vi "write positions to cvt or reload pico.vi"(8 "error in (no error)":errorcluster, 10 "Array":dbl[](array[numeric]), 11 "Picomotor8742dotNet in":refnum<class "Picomotor8742dotNet.lvclass">) -> (0 "error out":errorcluster, 2 "new command":string, 3 "Picomotor8742dotNet out":refnum<class "Picomotor8742dotNet.lvclass">)   [LabVIEW 2020, in "Picomotor8742dotNet.lvclass"]
uses:
  Picomotor8742dotNet.lvclass
  Picomotor8742dotNet.lvclass/Picomotor8742dotNet.ctl
  shared/CompressAndUpdate(Poly)/CompressAndUpdate(Numeric).vi
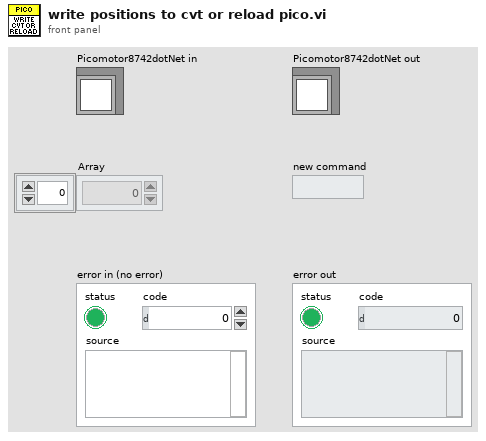
[diagram p1: front panel]
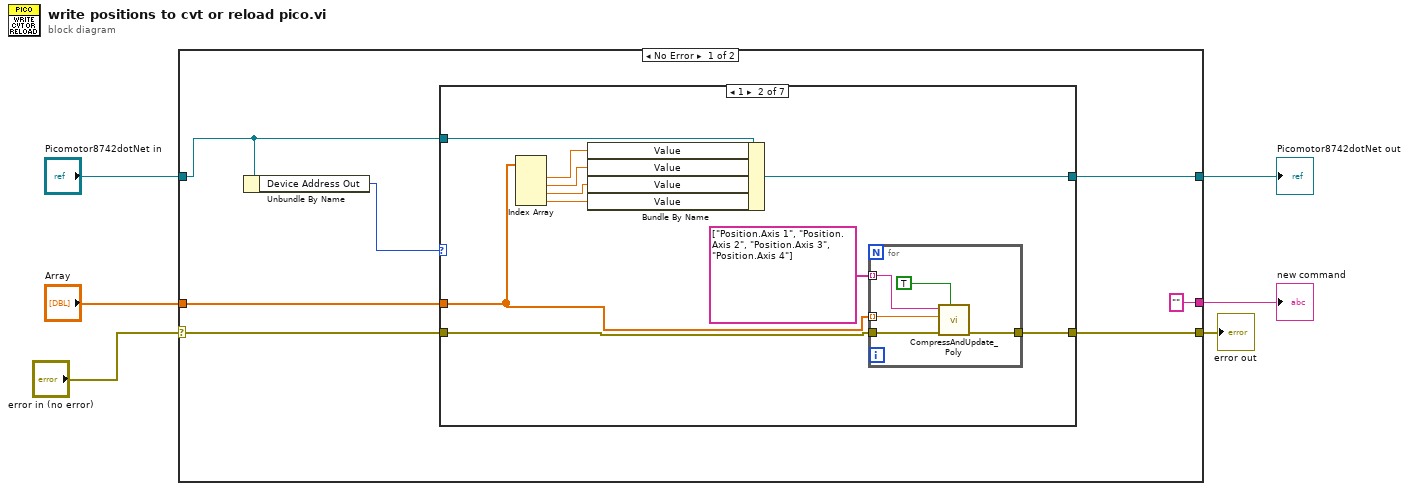
[diagram p0: block diagram]
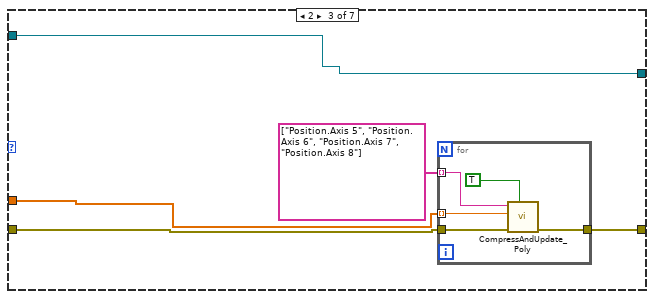
[diagram p3: hidden frame]
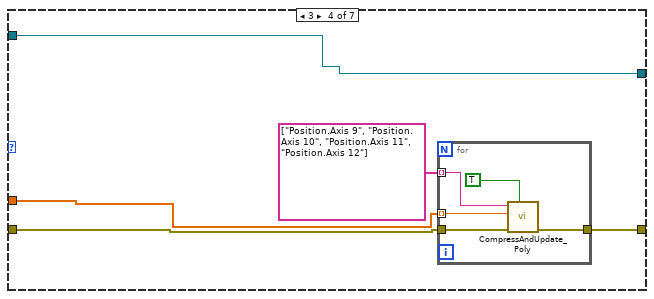
[diagram p4: hidden frame]
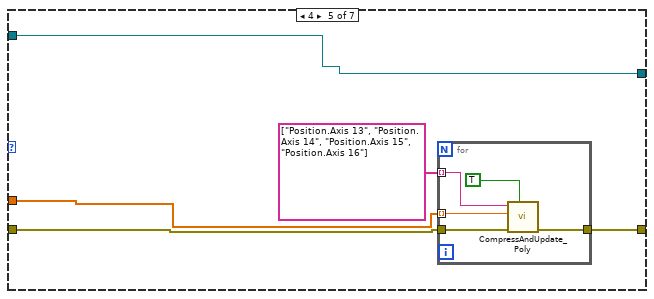
[diagram p5: hidden frame]
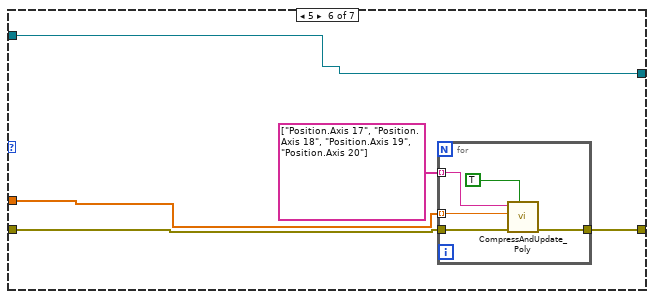
[diagram p6: hidden frame]
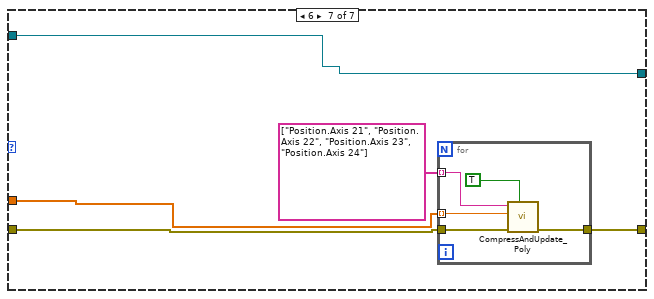
[diagram p7: hidden frame]
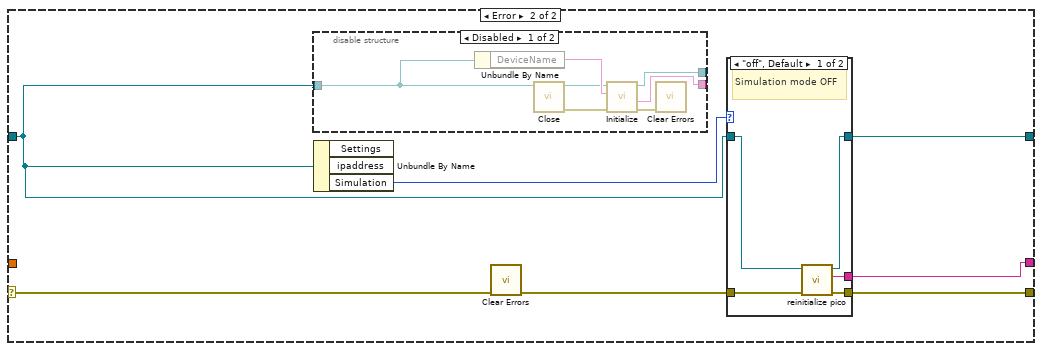
[diagram p8: hidden frame]
diagram:
  n1 = case shown="No Error" "error in (no error)" {
    selector: "error in (no error)" -> [w12 w86]
    tunnel: "Array" -> [w11 _]
    tunnel: [w13 w87] -> w2
    tunnel: "Picomotor8742dotNet in" -> [w8 w82]
    tunnel: [w10 w84] -> w4
    tunnel: ["" ("new command") w83] -> w5
    frame No Error {
      n2 = Unbundle By Name(w8) -> ("Device Address Out"=w7:i32)
      n3 = case shown="1" w7 {
        tunnel: [w14 w24 w34 w44 w54 w64 w74] -> w13
        tunnel: w12 -> [w14 w23 w33 w43 w53 w63 w73]
        tunnel: w11 -> [_ w18 w32 w42 w52 w62 w72]
        tunnel: [w15 w17 w31 w41 w51 w61 w71] -> w10
        tunnel: w8 -> [w15 w16 w31 w41 w51 w61 w71]
        frame 0, Default {
        }
        frame 1 {
          n4 = Index Array(array=w18) -> (element #1=w19:dbl, element #2=w20:dbl, element #3=w21:dbl, element #4=w22:dbl)  [unwired: 4 in]
          n5 = Bundle By Name(cluster=w16, "Value"=w19, "Value"=w20, "Value"=w21, "Value"=w22) -> (w17:refnum<class "Picomotor8742dotNet.lvclass">)
          n6 = for {
            tunnel: w18 -> [w28] mode=indexing
            tunnel: string[] ["Position.Axis 1", "Position.Axis 2", "Position.Axis 3", "Position.Axis 4"] -> [w29] mode=indexing
            tunnel: w23 -> [w27]
            tunnel: [w26] -> w24
            n7 = call-poly "CompressAndUpdate_Poly.vi"("force CVT update (false)"=TRUE ("force CVT update"), "error in"=w27, "Numeric"=w28, "command or variable name"=w29) -> ("error out"=w26:errorcluster)  [unwired: 7 in]
          }
        }
        frame 2 {
          n8 = for {
            tunnel: w32 -> [w38] mode=indexing
            tunnel: string[] ["Position.Axis 5", "Position.Axis 6", "Position.Axis 7", "Position.Axis 8"] -> [w39] mode=indexing
            tunnel: w33 -> [w37]
            tunnel: [w36] -> w34
            n9 = call-poly "CompressAndUpdate_Poly.vi"("force CVT update (false)"=TRUE ("force CVT update"), "error in"=w37, "Numeric"=w38, "command or variable name"=w39) -> ("error out"=w36:errorcluster)  [unwired: 7 in]
          }
        }
        frame 3 {
          n10 = for {
            tunnel: w42 -> [w48] mode=indexing
            tunnel: string[] ["Position.Axis 9", "Position.Axis 10", "Position.Axis 11", "Position.Axis 12"] -> [w49] mode=indexing
            tunnel: w43 -> [w47]
            tunnel: [w46] -> w44
            n11 = call-poly "CompressAndUpdate_Poly.vi"("force CVT update (false)"=TRUE ("force CVT update"), "error in"=w47, "Numeric"=w48, "command or variable name"=w49) -> ("error out"=w46:errorcluster)  [unwired: 7 in]
          }
        }
        frame 4 {
          n12 = for {
            tunnel: w52 -> [w58] mode=indexing
            tunnel: string[] ["Position.Axis 13", "Position.Axis 14", "Position.Axis 15", "Position.Axis 16"] -> [w59] mode=indexing
            tunnel: w53 -> [w57]
            tunnel: [w56] -> w54
            n13 = call-poly "CompressAndUpdate_Poly.vi"("force CVT update (false)"=TRUE ("force CVT update"), "error in"=w57, "Numeric"=w58, "command or variable name"=w59) -> ("error out"=w56:errorcluster)  [unwired: 7 in]
          }
        }
        frame 5 {
          n14 = for {
            tunnel: w62 -> [w68] mode=indexing
            tunnel: string[] ["Position.Axis 17", "Position.Axis 18", "Position.Axis 19", "Position.Axis 20"] -> [w69] mode=indexing
            tunnel: w63 -> [w67]
            tunnel: [w66] -> w64
            n15 = call-poly "CompressAndUpdate_Poly.vi"("force CVT update (false)"=TRUE ("force CVT update"), "error in"=w67, "Numeric"=w68, "command or variable name"=w69) -> ("error out"=w66:errorcluster)  [unwired: 7 in]
          }
        }
        frame 6 {
          n16 = for {
            tunnel: w72 -> [w78] mode=indexing
            tunnel: string[] ["Position.Axis 21", "Position.Axis 22", "Position.Axis 23", "Position.Axis 24"] -> [w79] mode=indexing
            tunnel: w73 -> [w77]
            tunnel: [w76] -> w74
            n17 = call-poly "CompressAndUpdate_Poly.vi"("force CVT update (false)"=TRUE ("force CVT update"), "error in"=w77, "Numeric"=w78, "command or variable name"=w79) -> ("error out"=w76:errorcluster)  [unwired: 7 in]
          }
        }
      }
    }
    frame Error {
      n18 = disable-structure shown="Disabled" {
        disable-tunnel: [w90 w95] -> _
        disable-tunnel: [w89 _] -> _
        disable-tunnel: w82 -> [w88 w95]
        frame Disabled {
          n19 = Unbundle By Name(w88) -> ("DeviceName"=w92:string)
          n20 = call-dynamic "Close.vi"("FakePressureController in"=w88) -> ("error out"=w93:errorcluster, "FakePressureController out"=w91:refnum<class "Picomotor8742dotNet.lvclass">)  [unwired: 7 in, 2 out]
          n21 = call-dynamic "Initialize.vi"("error in (no error)"=w93, "DeviceName"=w92, "Object in"=w91) -> ("error out"=w94:errorcluster, "new command(s)"=w89:string, "Object out"=w90:refnum<class "Picomotor8742dotNet.lvclass">)  [unwired: 5 in, 1 out]
          n22 = call <vilib>:"Clear Errors.vi"("error in (no error)"=w94) -> ()  [unwired: 5 in, 2 out]
        }
        frame Enabled {
        }
      }
      n23 = Unbundle By Name(w82) -> ("Simulation"=w81:enum16{"off", "on"})  [unwired: 2 out]
      n24 = call <vilib>:"Clear Errors.vi"("error in (no error)"=w86) -> ("error out"=w85:errorcluster)  [unwired: 5 in, 1 out]
      n25 = case shown="\"off\", Default" w81 {
        tunnel: w82 -> [w96 w102]
        tunnel: [w100 w102] -> w84
        tunnel: w85 -> [w98 w101]
        tunnel: [w99 w101] -> w87
        tunnel: [w97 _] -> w83
        frame "off", Default {
          # "Simulation mode OFF"
          n26 = call "reinitialize pico.vi"("error in (no error)"=w98, "Picomotor8742dotNet in"=w96) -> ("error out"=w99:errorcluster, "new command"=w97:string, "Picomotor8742dotNet out"=w100:refnum<class "Picomotor8742dotNet.lvclass">)  [unwired: 7 in]
        }
        frame "on" {
          # "Simulation mode ON"
        }
      }
    }
  }
  "new command" <- w5
  "Picomotor8742dotNet out" <- w4
  "error out" <- w2
